vi "UpdateRioDevice.vi"(9 "RIO Device":T2, 11 "References":T1) -> (0 "error out":errorcluster)   [LabVIEW 2014, in "FPGA Module editor node.lvclass"]
uses:
  FPGA Module editor node.lvclass
  <vilib>/userdefined/High Color/nirio_resource_hc.ctl
  <vilib>/NI/DCAF/Tag Editor Core/Table API/Table Manager/object ref.ctl
  <vilib>/NI/DCAF/Tag Editor Core/Configuration Editor/Classes/Engine Parent/Engine Parent Editor Node.lvclass
  <vilib>/NI/DCAF/Tag Editor Core/Configuration Editor/Classes/Module editor node/module editor node.lvclass
  module/configuration/FPGA Module configuration.lvclass
  module/configuration/FPGA Module configuration.lvclass/FPGA Module configuration.ctl
  module/configuration/Write RIO Device.vi
  <vilib>/NI/DCAF/Tag Editor Core/Configuration Editor/Classes/Module editor node/Read Module Configuration.vi
  <vilib>/NI/DCAF/Tag Editor Core/Configuration Editor/Classes/Module editor node/Write Module Configuration.vi
  <vilib>/NI/Tag Bus Module Framework/module configuration/TBM module configuration.lvclass
  <vilib>/NI/DCAF/Tag Editor Core/Table API/Table Manager/Table Manager.lvclass
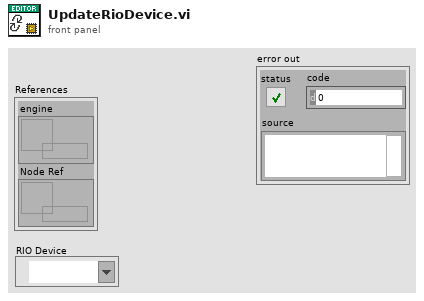
[diagram p1: front panel]
types:
  T1 = typedef "Table Manager.lvlib/Table Manager.lvclass/object ref.ctl" = cluster{"engine":refnum<data-value>, "Node Ref":refnum<data-value>}
  T2 = typedef "nirio_resource_hc.ctl" = tag
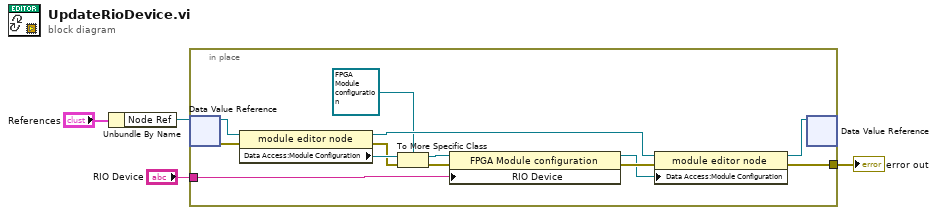
[diagram p0: block diagram]
diagram:
  n1 = Unbundle By Name("References") -> ("Node Ref"=w3:refnum<data-value>)
  n2 = in-place {
    in-place-border: [w8] -> w2
    in-place-border: "RIO Device" -> [w6]
    n3 = in-place-dvr #1(w3) -> (w17:refnum<class "module editor node.lvclass">, w7:errorcluster)
    n4 = property class="module editor node"(reference=w17, error in=w7) -> (reference out=w16:refnum<class "module editor node.lvclass">, error out=w11:errorcluster, "Data Access:Module Configuration"=w14:refnum<class "TBM module configuration.lvclass">)
    n5 = To More Specific Class(target class=refnum<class "FPGA Module configuration.lvclass"> refnum ("FPGA Module configuration"), reference=w14, error in=w11) -> (specific class reference=w13:refnum<class "FPGA Module configuration.lvclass">, error out=w10:errorcluster)
    n6 = property class="FPGA Module configuration"(reference=w13, error in=w10, "RIO Device"=w6) -> (reference out=w5:refnum<class "FPGA Module configuration.lvclass">, error out=w9:errorcluster)
    n7 = property class="module editor node"(reference=w16, error in=w9, "Data Access:Module Configuration"=w5) -> (reference out=w15:refnum<class "module editor node.lvclass">, error out=w8:errorcluster)
    n8 = in-place-dvr #1(w15) -> ()  [unwired: 2 out]
  }
  "error out" <- w2
